vi "Table Row.vi"(4 "Class (\"\")":string, 6 "Array of Cells (Empty Array)":string[](array[string]), 7 "Previous HTML in":string) -> (3 "HTML out":string)   [LabVIEW 2011]
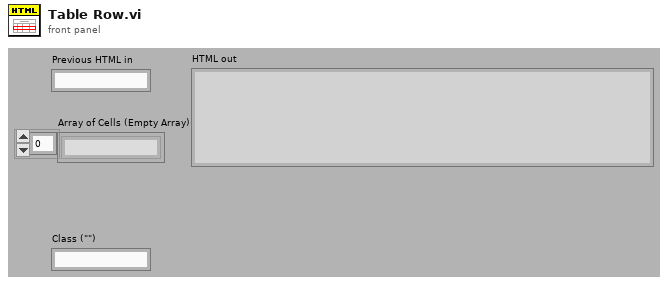
[diagram p1: front panel]
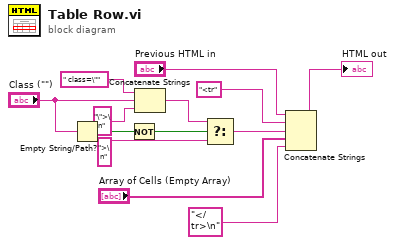
[diagram p0: block diagram]
diagram:
  n1 = Empty String/Path?(string/path="Class (\"\")") -> (empty?=w8:bool)
  n2 = Not(x=w8) -> (.not. x?=w1:bool)
  n3 = Concatenate Strings(" class=\"", "Class (\"\")", "\">\n") -> (w4:string)
  n4 = Select(t=w4, s=w1, f=">\n") -> (s? t:f=w2:string)
  n5 = Concatenate Strings("Previous HTML in", "<tr", w2, "Array of Cells (Empty Array)", "</tr>\n") -> (→"HTML out":string)
